vi "SensorFactory.vi"(8 "error in (no error)":errorcluster, 10 "Config":T1, 11 "SensorType":T2) -> (0 "error IO":errorcluster, 3 "Sensors.lvlib:Sensor.lvclass":refnum<class "Sensor.lvclass">)   [LabVIEW 2024, in "Sensors.lvlib"]
uses:
  Sensors.lvlib
  Controls/SensorType.ctl
  Controls/Config.ctl
  Sensor/Sensor.lvclass
  Simulated_Sensor/Simulated_Sensor.lvclass
  C:/Users/aheme/Documents/Dev/DEV_INFO/DEV_INFO/StockM/MyLabVIEW_Framework/Sensor/Sensor.lvclass
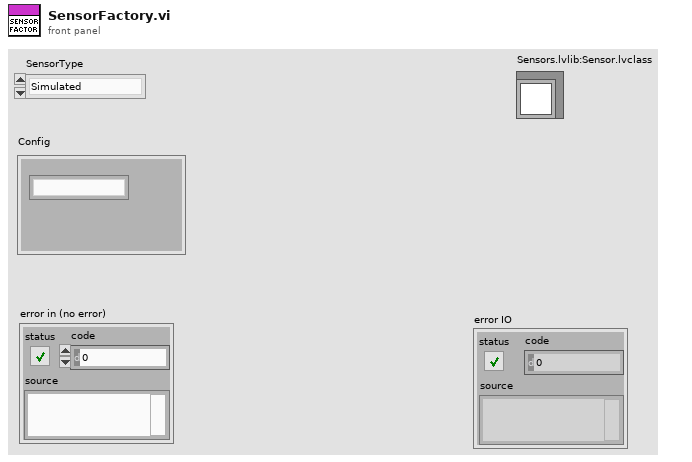
[diagram p1: front panel]
types:
  T1 = typedef "Sensors.lvlib/Config.ctl" = cluster{"String":string}
  T2 = typedef "Sensors.lvlib/SensorType.ctl" = enum16{"Simulated", "pH", "NPK"}
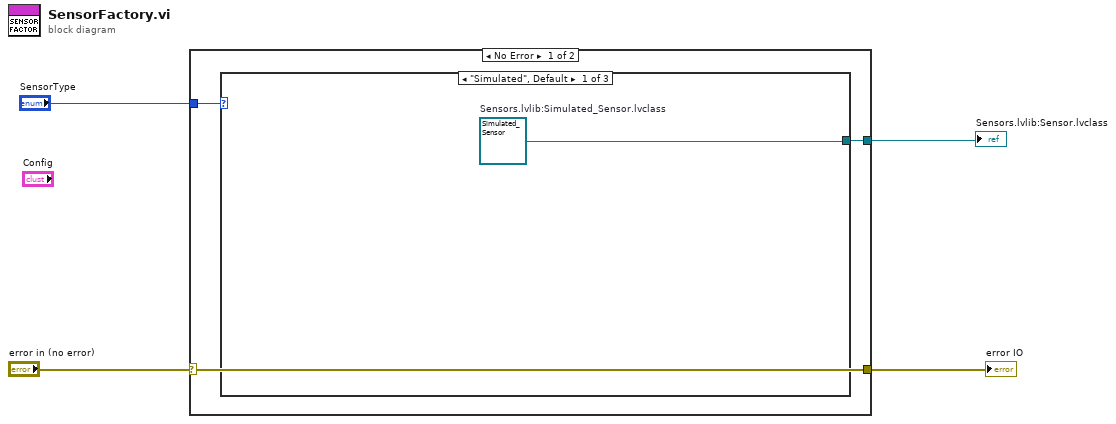
[diagram p0: block diagram]
diagram:
  n1 = case shown="No Error" "error in (no error)" {
    selector: "error in (no error)" -> [w7 w9]
    tunnel: [w7 w9] -> w3
    tunnel: "SensorType" -> [w6 _]
    tunnel: [w5 _] -> w1
    frame No Error {
      n2 = case shown="\"Simulated\", Default" w6 {
        tunnel: [w8 _ _] -> w5
        frame "Simulated", Default {
          w8 = refnum<class "Simulated_Sensor.lvclass"> refnum  # Sensors.lvlib:Simulated_Sensor.lvclass
        }
        frame "pH" {
        }
        frame "NPK" {
        }
      }
    }
    frame Error {
    }
  }
  "error IO" <- w3
  "Sensors.lvlib:Sensor.lvclass" <- w1
